vi "Get Movie Parameters (SubVI).vi"(11 "Parameters In":T1={"File REF"={"AVI REF"=refnum, "DBDE REF"=refnum}, "Frame Data"={"Width"=0, "Height"=0, "Frames Per Second"=0, "Codec"=""}, "File Type"="", "Experiment Mode"=enum."Replay", "Movie File Path"=path "D:/Movies Formatted on November 5th 2015/Clip (2) Formatted.raw"}) -> (3 "Parameters Out":T1={"File REF"={"AVI REF"=refnum, "DBDE REF"=refnum}, "Frame Data"={"Width"=0, "Height"=0, "Frames Per Second"=0, "Codec"=""}, "File Type"="", "Experiment Mode"=enum."Live", "Movie File Path"=path "D:/Movies Formatted on November 5th 2015/Clip (2) Formatted.raw"})   [LabVIEW 2020]
uses:
  Controls (HOST)/IMAQ Parameters.ctl
  Controls (HOST)/File REF.ctl
  <vilib>/vision/Avi.llb/IMAQ AVI2 Refnum.ctl
  Controls (HOST)/Experiment Mode.ctl
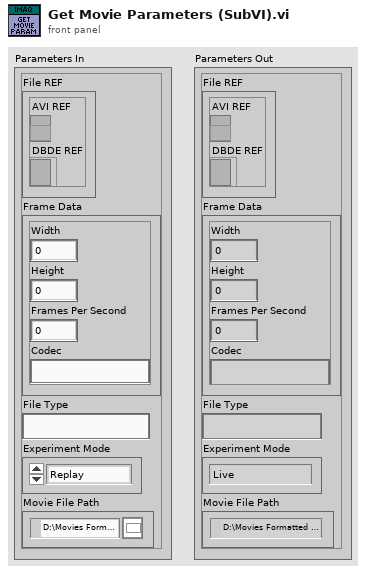
[diagram p1: front panel]
types:
  T1 = typedef "IMAQ Parameters.ctl" = cluster{"File REF":T2, "Frame Data":cluster{"Width":u32, "Height":u32, "Frames Per Second":u32, "Codec":string}, "File Type":string, "Experiment Mode":T4, "Movie File Path":path}
  T2 = typedef "File REF.ctl" = cluster{"AVI REF":T3, "DBDE REF":refnum<file>}
  T3 = typedef "IMAQ AVI2 Refnum.ctl" = refnum<k20>
  T4 = typedef "Experiment Mode.ctl" = enum16{"Live", "Replay"}
  T5 = cluster{"Width":u32, "Height":u32, "Frames Per Second":u32, "Codec":string}
  T6 = enum16{"big-endian, network order", "native, host order", "little-endian"}
  T7 = cluster{"Width":u32, "Height":u32, "Frames Per Second":u32, "Codec":string, "Has Data":bool}
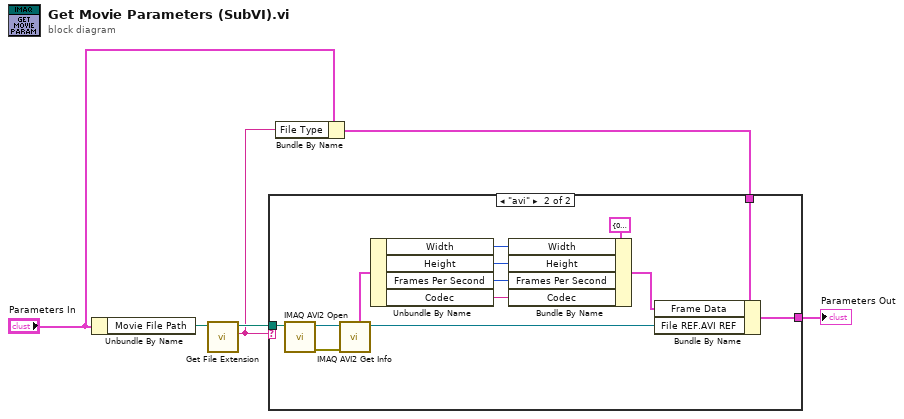
[diagram p0: block diagram]
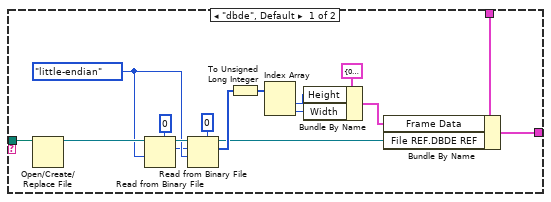
[diagram p2: hidden frame]
diagram:
  n1 = Unbundle By Name("Parameters In") -> ("Movie File Path"=w5:path)
  n2 = call <vilib>:"Get File Extension.vi"("file"=w5) -> ("lowercase file extension"=w3:string, "dup file"=w6:path)  [unwired: 6 in, 3 out]
  n3 = Bundle By Name(cluster="Parameters In", "File Type"=w3) -> (w2:T1)
  n4 = case shown="\"avi\"" w3 {
    tunnel: w6 -> [w22 w33]
    tunnel: [w8 w25] -> w1
    tunnel: w2 -> [w7 w26]
    frame "dbde", Default {
      w15 = T6."little-endian" ("byte order (0:big-endian, network order)")
      n5 = Open/Create/Replace File(file path (use dialog)=w22) -> (refnum out=w21:refnum<file>)  [unwired: 5 in, 2 out]
      n6 = Read from Binary File(5:0 ("count (1)"), 9:w15, 11:w21) -> (2:w14:i32, 3:w20:refnum<file>)  [unwired: 3 in, 2 out]
      n7 = Read from Binary File(5:u64 0 ("count (1)"), 9:w15, 10:w14, 11:w20) -> (2:w12:u64[], 3:w9:refnum<file>)  [unwired: 2 in, 2 out]
      n8 = To Unsigned Long Integer(number=w12) -> (unsigned 32bit integer=w16:u32[])
      n9 = Index Array(array=w16) -> (element #1=w18:u32, element #2=w17:u32)  [unwired: 2 in]
      n10 = Bundle By Name(cluster=T5 {"Width"=0, "Height"=0, "Frames Per Second"=0, "Codec"=""} ("Frame Data"), "Height"=w18, "Width"=w17) -> (w10:T5)
      n11 = Bundle By Name(cluster=w7, "Frame Data"=w10, "File REF.DBDE REF"=w9) -> (w8:T1)
    }
    frame "avi" {
      n12 = call "IMAQ AVI2 Open"("AVI File Path"=w33) -> ("error out"=w35:errorcluster, "AVI Refnum"=w34:T3)  [unwired: 9 in]
      n13 = call "IMAQ AVI2 Get Info"("error in (no error)"=w35, "AVI Refnum"=w34) -> ("AVI Refnum (duplicate)"=w23:T3, "Frame Data"=w31:T7)  [unwired: 5 in, 3 out]
      n14 = Unbundle By Name(w31) -> ("Width"=w30:u32, "Height"=w29:u32, "Frames Per Second"=w28:u32, "Codec"=w27:string)
      n15 = Bundle By Name(cluster=T5 {"Width"=0, "Height"=0, "Frames Per Second"=0, "Codec"=""} ("Frame Data"), "Width"=w30, "Height"=w29, "Frames Per Second"=w28, "Codec"=w27) -> (w24:T5)
      n16 = Bundle By Name(cluster=w26, "Frame Data"=w24, "File REF.AVI REF"=w23) -> (w25:T1)
    }
  }
  "Parameters Out" <- w1
